vi "Medidas de convercion andy camargo.vi"() -> ()   [LabVIEW 2013]
panel:
  out "RESULTADO KL-MM":dbl format="%#13_13g"
  in  "Boton de km-mm":bool
  in  "CANTIDAD DE KL-MM":dbl
  out "CANTIDAD MILI-CENTIM":dbl
  in  "Boton mili-cm":bool
  in  "CANTIDAD MILI-CENTIM":dbl
  out "RESULTADO M-K":dbl
  in  "CANTIDAD M-K":dbl
  in  "Boton m-k":bool
  out "RESULTADO cm-m":dbl
  in  "Boton cm-m":bool
  in  "CANTIDAD cm-m":dbl
  # "UNIVERSIDAD DE CUNDINAMARCA\nINGENIERIA DE SISTEMAS X\nELECTIVA PROFECIONAL IV\nANDY LEANDRO CAMARGO"
  # "kilometros-milimetros"
  # "milimetros-kilometros"
  # "metro-kilometro"
  # "kilometro-metro"
  # "metro-centimetros"
  # "centimetro-metros"
  # "milimetro-centimetro"
  # "centimetro-milimetro"
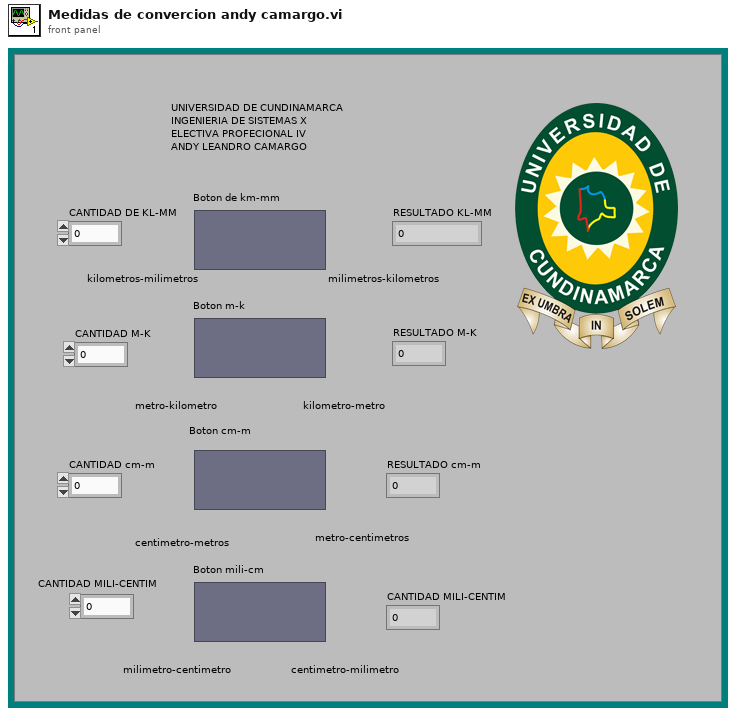
[diagram p1: front panel]
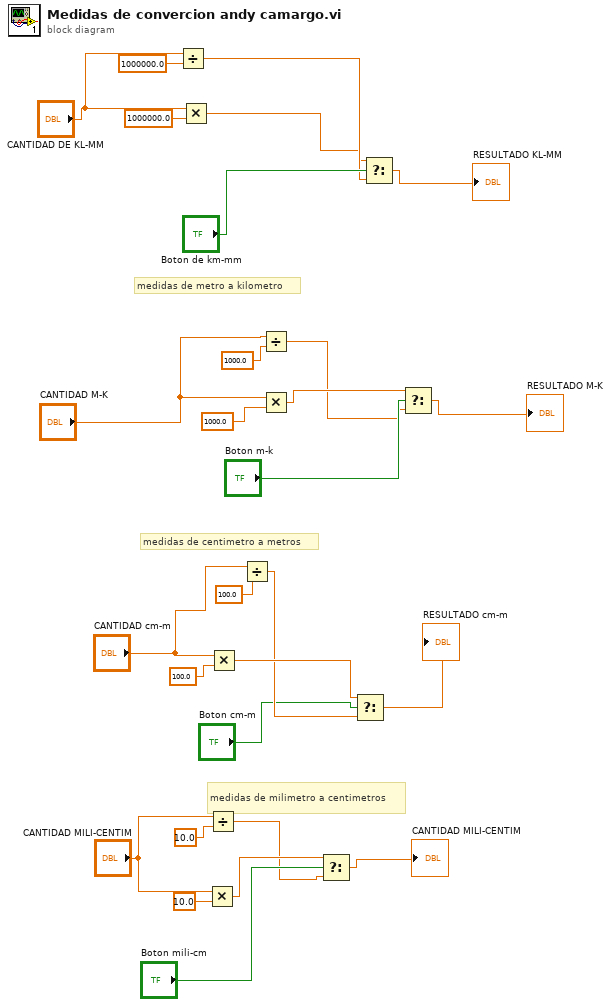
[diagram p0: block diagram]
diagram:
  # "medidas de milimetro a centimetros"
  # "medidas de centimetro a metros"
  # "medidas de metro a kilometro"
  n1 = Divide(x="CANTIDAD DE KL-MM", y=1000000.0) -> (x/y=w5:dbl)
  n2 = Multiply(x="CANTIDAD DE KL-MM", y=1000000.0) -> (x*y=w4:dbl)
  n3 = Multiply(x="CANTIDAD MILI-CENTIM", y=10.0) -> (x*y=w9:dbl)
  n4 = Divide(x="CANTIDAD MILI-CENTIM", y=10.0 ("x")) -> (x/y=w8:dbl)
  n5 = Multiply(x="CANTIDAD cm-m", y=100.0 ("x")) -> (x*y=w27:dbl)
  n6 = Divide(x="CANTIDAD cm-m", y=100.0 ("x/y")) -> (x/y=w24:dbl)
  n7 = Divide(x="CANTIDAD M-K", y=1000.0 ("x")) -> (x/y=w16:dbl)
  n8 = Multiply(x="CANTIDAD M-K", y=1000.0) -> (x*y=w17:dbl)
  n9 = Select(t=w9, s="Boton mili-cm", f=w8) -> (s? t:f=→"CANTIDAD MILI-CENTIM":dbl)
  n10 = Select(t=w27, s="Boton cm-m", f=w24) -> (s? t:f=→"RESULTADO cm-m":dbl)
  n11 = Select(t=w4, s="Boton de km-mm", f=w5) -> (s? t:f=→"RESULTADO KL-MM":dbl)
  n12 = Select(t=w17, s="Boton m-k", f=w16) -> (s? t:f=→"RESULTADO M-K":dbl)
